vi "tm460_dcimgreader.vi"() -> ()   [LabVIEW 2023, in "HamamatsuCam.lvlib" / "HamamatsuCam.lvclass"]
uses:
  HamamatsuCam/HamamatsuCam/HamamatsuCam.lvclass
panel:
  out "Current Frame":i32
  out "Error Out":errorcluster
  out "Image":u16[][](graph)
  out "Timestamp":dbl
  out "Total":i32
  in  "DCIMG Path":path
  # "This is an example of how to read\nthe images within a DCIMG file."
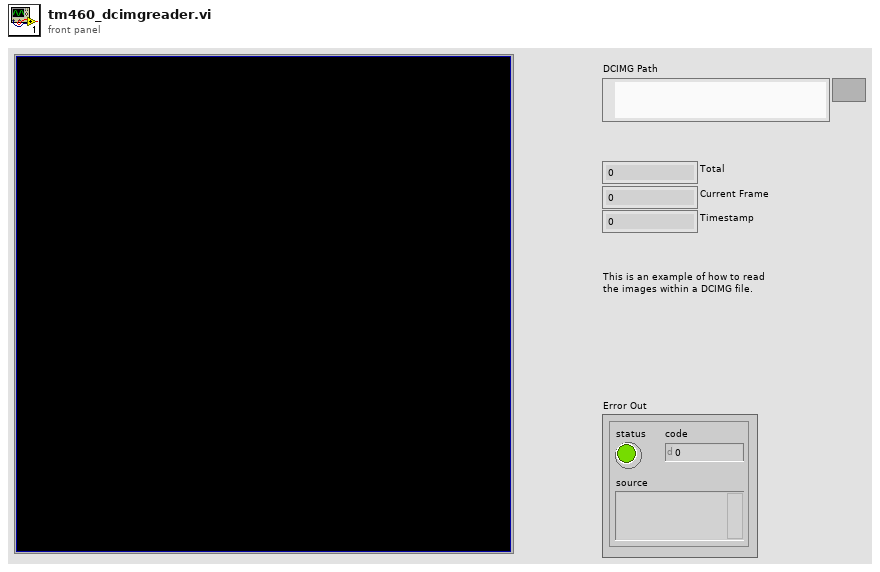
[diagram p1: front panel]
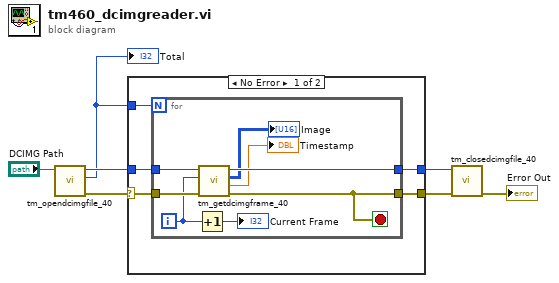
[diagram p0: block diagram]
diagram:
  n1 = call "tm_opendcimgfile_40.vi"("Path"="DCIMG Path") -> ("error out"=w4:errorcluster, "Total Frames"=w5:i32, "File Handle"=w6:u32)  [unwired: 8 in]
  "Total" <- w5
  n2 = case shown="No Error" w4 {
    selector: w4 -> [w10 w21]
    tunnel: w6 -> [w12 w22]
    tunnel: w5 -> [w11 _]
    tunnel: [w9 w22] -> w2
    tunnel: [w8 w21] -> w3
    frame No Error {
      n3 = for {
        N: w11 -> [_]
        tunnel: w12 -> [w20]
        tunnel: w10 -> [w19]
        tunnel: [w15] -> w8
        tunnel: [w18] -> w9
        i -> [w14]
        stop <- w15 stop-if-true
        n4 = Increment(x=w14) -> (x+1=→"Current Frame":i32)
        n5 = call "tm_getdcimgframe_40.vi"("error in (no error)"=w19, "Frame Index"=w14, "File Handle in"=w20) -> ("error out"=w15:errorcluster, "Timestamp"=→"Timestamp":dbl, "Data"=→"Image":u16[][], "File Handle out"=w18:u32)  [unwired: 5 in]
      }
    }
    frame Error {
    }
  }
  n6 = call "tm_closedcimgfile_40.vi"("error in (no error)"=w3, "File Handle"=w2) -> ("error out"=→"Error Out":errorcluster)  [unwired: 9 in]
